vi "Finalize Localization Data (SubVI).vi"(8 "Avg rcy":dbl, 9 "Avg rcx":dbl, 10 "Avg lcy":dbl, 11 "Avg lcx":dbl) -> (1 "Heading":dbl, 2 "Center Y":dbl, 3 "Center X":dbl)   [LabVIEW 2015]
uses:
  <vilib>/express/express arith-compare/Formula/XNode/ExpressFormulaBlockNode.xnode
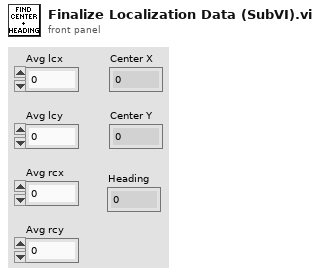
[diagram p1: front panel]
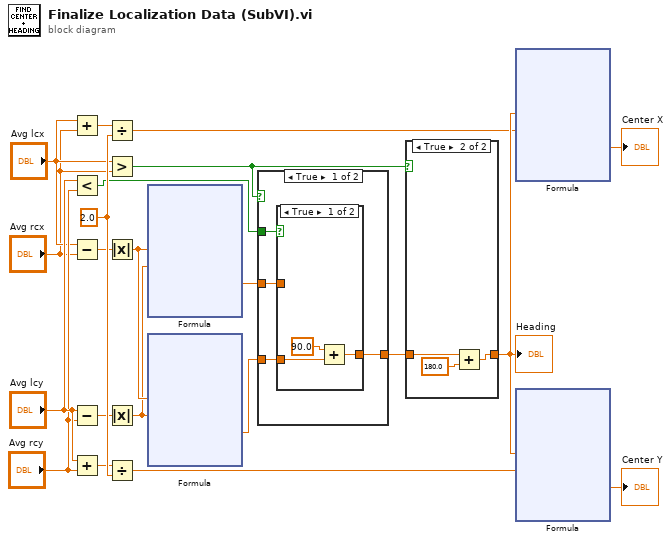
[diagram p0: block diagram]
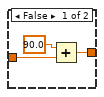
[diagram p4: hidden frame]
diagram:
  w21 = 2.0
  n1 = Add(x="Avg lcx", y="Avg rcx") -> (x+y=w20:dbl)
  n2 = Less?(x="Avg lcy", y="Avg rcy") -> (x < y?=w12:bool)
  n3 = Subtract(x="Avg lcx", y="Avg rcx") -> (x-y=w18:dbl)
  n4 = Subtract(x="Avg lcy", y="Avg rcy") -> (x-y=w17:dbl)
  n5 = Add(x="Avg lcy", y="Avg rcy") -> (x+y=w19:dbl)
  n6 = Divide(x=w20, y=w21) -> (x/y=w4:dbl)
  n7 = Greater?(x="Avg lcx", y="Avg rcx") -> (0:w1:bool)
  n8 = Absolute Value(x=w18) -> (abs(x)=w16:dbl)
  n9 = Absolute Value(x=w17) -> (abs(x)=w15:dbl)
  n10 = Divide(x=w19, y=w21) -> (x/y=w6:dbl)
  n11 = xnode "Formula"("Width"=w16, "Depth"=w15) -> ("Result"=w11:dbl)  [unwired: 1 in, 1 out]
  n12 = xnode "Formula"("Width"=w16, "Depth"=w15) -> ("Result"=w10:dbl)  [unwired: 1 in, 1 out]
  n13 = case shown="True" w1 {
    tunnel: w12 -> [w25 w33]
    tunnel: w11 -> [w24 w32]
    tunnel: w10 -> [w23 w31]
    tunnel: [w22 w30] -> w7
    frame True {
      n14 = case shown="True" w25 {
        tunnel: [w26 w29] -> w22
        tunnel: w24 -> [_ w29]
        tunnel: w23 -> [w27 _]
        frame True {
          n15 = Add(x=90.0, y=w27) -> (x+y=w26:dbl)
        }
        frame False {
        }
      }
    }
    frame False {
      n16 = case shown="True" w33 {
        tunnel: [w34 w37] -> w30
        tunnel: w32 -> [_ w37]
        tunnel: w31 -> [w35 _]
        frame False {
          n17 = Add(x=90.0, y=w35) -> (x+y=w34:dbl)
        }
        frame True {
        }
      }
    }
  }
  n18 = case shown="True" w1 {
    tunnel: w7 -> [w38 w41]
    tunnel: [w38 w39] -> w5
    frame False {
    }
    frame True {
      n19 = Add(x=w41, y=180.0) -> (x+y=w39:dbl)
    }
  }
  "Heading" <- w5
  n20 = xnode "Formula"("Heading"=w5, "midpointX"=w4) -> ("Result"=→"Center X":dbl)  [unwired: 1 in, 1 out]
  n21 = xnode "Formula"("Heading"=w5, "midpointY"=w6) -> ("Result"=→"Center Y":dbl)  [unwired: 1 in, 1 out]
